vi "Spammer.vi"() -> ()   [LabVIEW 2016]
uses:
  <vilib>/ORNL/CSEISMIC DDS/CSEISMIC DDS Base/Data Types/Controls/DeviceClass Selector.ctl
  <vilib>/ORNL/CSEISMIC DDS/CSEISMIC DDS Base/CSEISMIC DDS.lvclass/CSEISMIC DDS.ctl
  <vilib>/ORNL/CSEISMIC DDS/CSEISMIC DDS Base/Data Types/IED_Status.ctl
  <vilib>/ORNL/CSEISMIC DDS/CSEISMIC DDS Base/Data Types/Controls/DeviceID.ctl
  <vilib>/ORNL/CSEISMIC DDS/CSEISMIC DDS Base/Data Types/Controls/Timestamp.ctl
  <vilib>/ORNL/CSEISMIC DDS/CSEISMIC DDS Base/Accessors/Write DDS Reference.vi
  <vilib>/ORNL/CSEISMIC DDS/CSEISMIC DDS Base/Accessors/Read DDS Reference.vi
  <vilib>/ORNL/CSEISMIC DDS/DDS Writer/DDS Writer.lvclass
  C:/Program Files (x86)/National Instruments/LabVIEW 2016/vi.lib/ORNL/CSEISMIC DDS/CSEISMIC DDS Base/CSEISMIC DDS.lvclass
  <vilib>/ORNL/CSEISMIC DDS/CSEISMIC DDS Base/Error Handler.vi
  <vilib>/ORNL/CSEISMIC DDS/CSEISMIC DDS Base/CSEISMIC DDS.lvclass
panel:
  in  "DeviceClass":T1=256 format="%04x" items=["Invalid"=0, "IED"=256, "DER"=512, "Relay"=768, "Meter"=1024, "Load"=1280, "Forecast"=1536, "Price"=1792, "Energy Storage"=513, "PV"=514, "Generator"=515, "Smart Relay"=769, "PCC"=770, "Smart Meter"=1025, "PMU"=1026, "HVAC"=1281]
  in  "stop":bool
  out "error out":errorcluster
  in  "error in":errorcluster
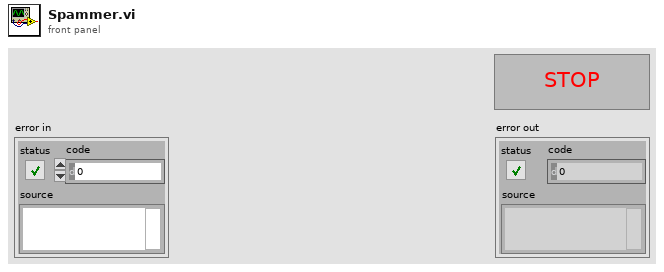
[diagram p1: front panel]
types:
  T1 = typedef "CSEISMIC DDS.lvlib/CSEISMIC DDS.lvclass/DeviceClass Selector.ctl" = u16
  T2 = typedef "CSEISMIC DDS.lvlib/CSEISMIC DDS.lvclass/IED_Status.ctl" = cluster{"DeviceID":T3, "Timestamp":T4, "MicrogridID":u8, "Active":bool, "Inactive":bool, "Error":i32, "Fault":bool, "ErrorString":string}
  T3 = typedef "CSEISMIC DDS.lvlib/CSEISMIC DDS.lvclass/DeviceID.ctl" = string
  T4 = typedef "CSEISMIC DDS.lvlib/CSEISMIC DDS.lvclass/Timestamp.ctl" = cluster{"Seconds":u64, "Remainder":u64}
  T5 = typedef "LVStringsAndValuesArrayTypeDef_U16.ctl" = cluster{"String":string, "Value":u16}[]
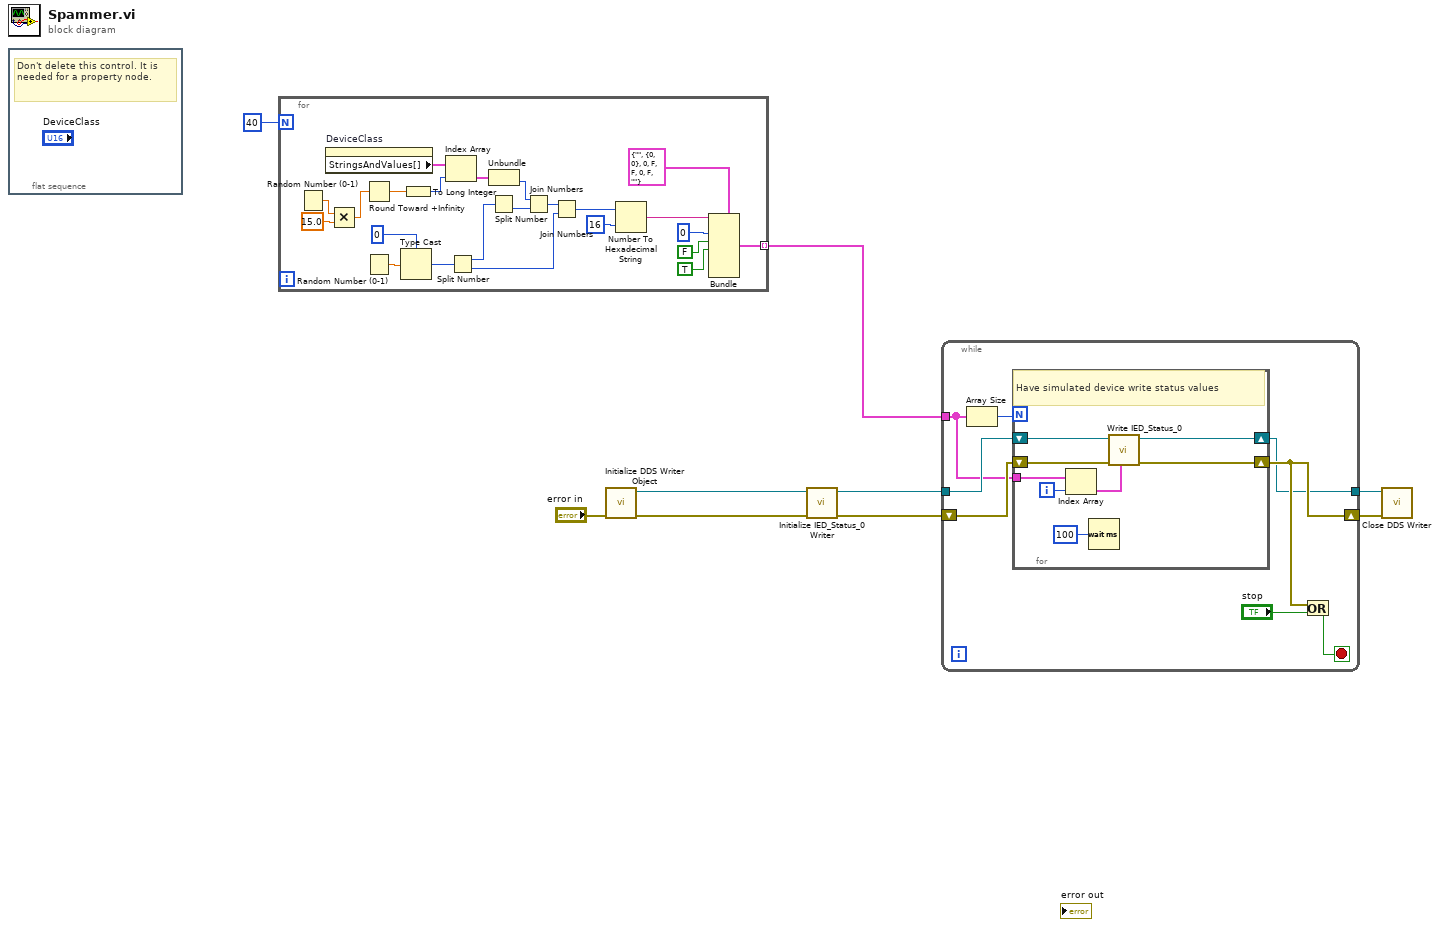
[diagram p0: block diagram]
diagram:
  n1 = flat-sequence {
    frame #0 {
      # "Don't delete this control. It is needed for a property node."
    }
  }
  n2 = for {
    N: 40 -> [_]
    tunnel: [w16] -> w8 mode=indexing
    n3 = Random Number (0-1)() -> (number: 0 to 1=w31:dbl)
    n4 = property on="DeviceClass" class="Ring (strict)"() -> ("StringsAndValues[]"=w28:T5)  [unwired: 2 in, 2 out]
    n5 = Multiply(x=w31, y=15.0) -> (x*y=w29:dbl)
    n6 = Round Toward +Infinity(x=w29) -> (ceil(x): smallest int >= x=w27:dbl)
    n7 = Random Number (0-1)() -> (number: 0 to 1=w24:dbl)
    n8 = Type Cast(type=u64 0 ("x"), x=w24) -> (*(type *) &x=w22:u64)
    n9 = To Long Integer(number=w27) -> (32bit integer=w26:i32)
    n10 = Index Array(array=w28, index=w26) -> (element=w25:cluster{"String":string, "Value":u16})
    n11 = Split Number(x=w22) -> (hi(x)=w21:u32, lo(x)=w18:u32)
    n12 = Unbundle(w25) -> ("Value"=w20:u16)  [unwired: 1 out]
    n13 = Split Number(x=w21) -> (lo(x)=w19:u16)  [unwired: 1 out]
    n14 = Join Numbers(hi=w20, lo=w19) -> ((hi.lo)=w32:u32)
    n15 = Join Numbers(hi=w32, lo=w18) -> ((hi.lo)=w12:u64)
    n16 = Number To Hexadecimal String(1:i16 16 ("width (-)"), 2:w12) -> (0:w10:string)
    n17 = Bundle(cluster=T2 {"DeviceID"="", "Timestamp"={"Seconds"=0, "Remainder"=0}, "MicrogridID"=0, "Active"=FALSE, "Inactive"=FALSE, "Error"=0, "Fault"=FALSE, "ErrorString"=""} ("Status_IED"), "DeviceID"=w10, "MicrogridID"=u8 0, "Active"=FALSE ("Inactive"), "Inactive"=TRUE ("Active")) -> (w16:T2)  [unwired: 4 in]
  }
  n18 = call <vilib>:"Initialize DDS Writer Object.vi"("error in"="error in") -> ("error out"=w5:errorcluster, "DDS Writer out"=w6:refnum<class "DDS Writer.lvclass">)  [unwired: 9 in]
  n19 = call <vilib>:"Initialize IED_Status_0 Writer.vi"("error in"=w5, "DDS Writer in"=w6) -> ("error out"=w4:errorcluster, "DDS Writer out"=w3:refnum<class "DDS Writer.lvclass">)  [unwired: 8 in]
  n20 = while {
    shift-right: [w37] -> w1
    shift-left: w4 -> [w40]
    tunnel: w3 -> [w36]
    tunnel: [w35] -> w2
    tunnel: w8 -> [w33]
    stop <- w39 stop-if-true
    n21 = Array Size(array=w33) -> (size(s)=w34:i32)
    n22 = for {
      N: w34 -> [_]
      shift-right: [w44] -> w35
      shift-left: w36 -> [w47]
      shift-right: [w45] -> w37
      shift-left: w40 -> [w46]
      tunnel: w33 -> [w43]
      i -> [w42]
      # "Have simulated device write status values"
      n23 = Index Array(array=w43, index=w42) -> (element=w41:T2)
      n24 = Wait (ms)(milliseconds to wait=u32 100) -> ()  [unwired: 1 out]
      n25 = call <vilib>:"Write IED_Status_0.vi"("IED_Status"=w41, "error in"=w46, "DDS Writer in"=w47) -> ("error out"=w45:errorcluster, "DDS Writer out"=w44:refnum<class "DDS Writer.lvclass">)  [unwired: 7 in]
    }
    n26 = Or(x=w37, y="stop") -> (x .or. y?=w39:bool)
  }
  n27 = call <vilib>:"Close DDS Writer.vi"("error in"=w1, "DDS Writer in"=w2) -> ()  [unwired: 9 in, 1 out]
